vi "ASCII string to Hex string.vi"(4 "ASCII string":string) -> (1 "hex String":string)   [LabVIEW 2013]
doc: "Prepends < and postpends > to a string."
panel:
  # "hex display"
  # "normal display"
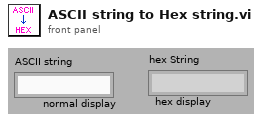
[diagram p1: front panel]
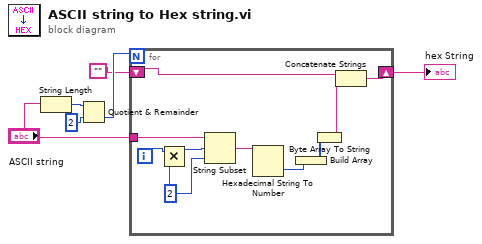
[diagram p0: block diagram]
diagram:
  n1 = String Length(string="ASCII string") -> (length=w4:i32)
  n2 = Quotient & Remainder(x=w4, y=2) -> (floor(x/y)=w2:i32)  [unwired: 1 out]
  n3 = for {
    N: w2 -> [_]
    shift-right: [w15] -> w6
    shift-left: "" -> [w16]
    tunnel: "ASCII string" -> [w11]
    i -> [w14]
    w13 = 2 ("length (rest)")
    n4 = Multiply(x=w14, y=w13) -> (x*y=w12:i32)
    n5 = String Subset(string=w11, offset (0)=w12, length (rest)=w13) -> (substring=w10:string)
    n6 = Hexadecimal String To Number(string=w10) -> (number=w9:u32)  [unwired: 3 out]
    n7 = Build Array(w9) -> (w8:u32[])
    n8 = Byte Array To String(unsigned byte array=w8) -> (string=w7:string)
    n9 = Concatenate Strings(w16, w7) -> (w15:string)
  }
  "hex String" <- w6
